vi "Initialize From Settings.vi"(8 "error in (no error)":errorcluster, 10 "settings":cluster{"key":string, "value":string}[](array[cluster]), 11 "RDMA Plugin Configuration in":refnum<class "RDMA Plugin Configuration.lvclass">) -> (0 "error out":errorcluster, 3 "RDMA Plugin Configuration out":refnum<class "RDMA Plugin Configuration.lvclass">)   [LabVIEW 2020, in "RDMA.lvlib" / "RDMA Plugin Configuration.lvclass"]
uses:
  RDMA Plugin Configuration.lvclass
  Plugin Settings.ctl
  RDMA Plugin Configuration.lvclass/RDMA Plugin Configuration.ctl
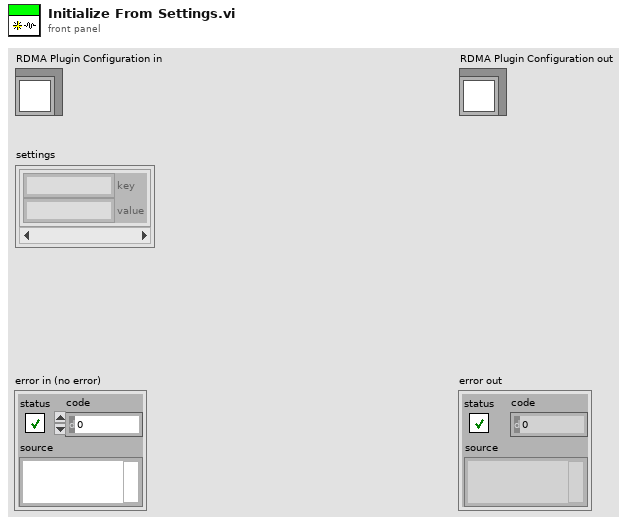
[diagram p1: front panel]
types:
  T1 = typedef "RDMA.lvlib/RDMA Plugin Configuration.lvclass/Plugin Settings.ctl" = cluster{"initialization timeout s":dbl}
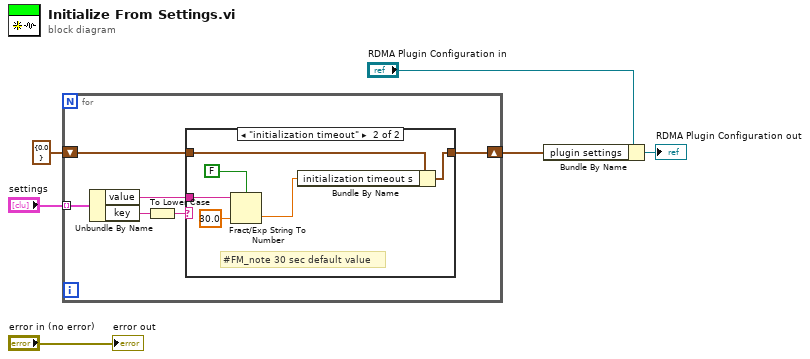
[diagram p0: block diagram]
diagram:
  n1 = for {
    tunnel: "settings" -> [w12] mode=indexing
    shift-right: [w7] -> w1
    shift-left: T1 {"initialization timeout s"=0.0} ("plugin settings") -> [w11]
    n2 = Unbundle By Name(w12) -> ("value"=w10:string, "key"=w9:string)
    n3 = To Lower Case(string=w9) -> (all lower case string=w8:string)
    n4 = case shown="\"initialization timeout\"" w8 {
      tunnel: w11 -> [w13 w19]
      tunnel: w10 -> [_ w18]
      tunnel: [w13 w15] -> w7
      frame Default {
      }
      frame "initialization timeout" {
        # "#FM_note 30 sec default value"
        n5 = Fract/Exp String To Number(use system decimal point (T)=FALSE, string=w18, default (0 dbl)=30.0 ("default (0 DBL)")) -> (number=w16:dbl)  [unwired: 1 in, 1 out]
        n6 = Bundle By Name(cluster=w19, "initialization timeout s"=w16) -> (w15:T1)
      }
    }
  }
  n7 = Bundle By Name(cluster="RDMA Plugin Configuration in", "plugin settings"=w1) -> (→"RDMA Plugin Configuration out":refnum<class "RDMA Plugin Configuration.lvclass">)
  "error out" <- "error in (no error)"
